vi "Header Footer Alignment.vi"(3 "H/F Alignment":T1) -> (0 "Vertical Alignement":T2, 1 "Horizontal Alignment":T3)   [LabVIEW 2012]
doc: "Version 1.0\nDeveloped by Jean-Marc Simard\nCopyright © 2010, Exaprom Inc.\nAll rights reserved.\nLicense: BSD\n\nWith iTextSharp 4.1.6 (http://itextsharp.sourceforge.net)\nunder Mozilla Public License Version 1.1\n(http://www.mozilla.org/MPL/MPL-1.1.html)"
uses:
  Controls/Header footer horiz alignment.ctl
  Controls/Cell Vertical alignment.ctl
  Controls/H F Alignment.ctl
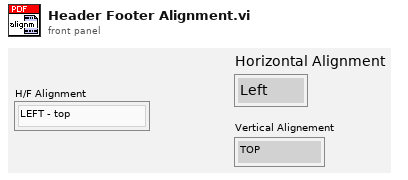
[diagram p1: front panel]
types:
  T1 = typedef "H F Alignment.ctl" = enum16{"LEFT - top", "LEFT - middle", "LEFT - bottom", "CENTER - top", "CENTER - middle", "CENTER - bottom", "RIGHT - top", "RIGHT - middle", "RIGHT - bottom", ""}
  T2 = typedef "Cell Vertical alignment.ctl" = enum16{"TOP", "MIDDLE", "BOTTOM"}
  T3 = typedef "Header footer horiz alignment.ctl" = enum16{"Left", "Center", "Right"}
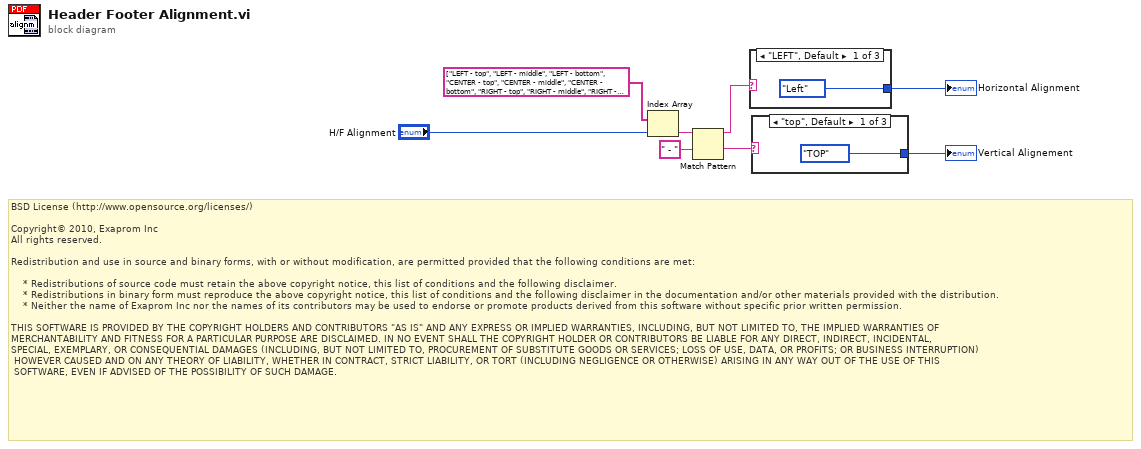
[diagram p0: block diagram]
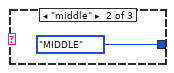
[diagram p2: hidden frame]
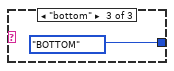
[diagram p3: hidden frame]
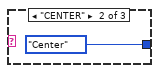
[diagram p4: hidden frame]
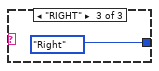
[diagram p5: hidden frame]
diagram:
  # "BSD License (http://www.opensource.org/licenses/)\n\nCopyright© 2010, Exaprom Inc\nAll rights reserved.\n\nRedistribution and use in source and binary forms, with or without modification, are permitted provided that the following conditions are met:\n\n    * Redistributions of source code must retain the above copyright notice, this list of conditions and the following disclaimer.\n    * Redistributions in binary form must reproduce the above copyright notice, this list of conditions and the following disclaimer in the documentation and/or other materials provided with the distribution.\n    * Neither the name of Exaprom Inc nor the names of its contributors may be used to endorse or promote products derived from this software without specific prior written permission.\n\nTHIS SOFTWARE IS PROVIDED BY THE COPYRIGHT HOLDERS AND CONTRIBUTORS \"AS IS\" AND ANY EXPRESS OR IMPLIED WARRANTIES, INCLUDING, BUT NOT LIMITED TO, THE IMPLIED WARRANTIES OF \nMERCHANTABILITY AND FITNESS FOR A PARTICULAR PURPOSE ARE DISCLAIMED. IN NO EVENT SHALL THE COPYRIGHT HOLDER OR CONTRIBUTORS BE LIABLE FOR ANY DIRECT, INDIRECT, INCIDENTAL,\nSPECIAL, EXEMPLARY, OR CONSEQUENTIAL DAMAGES (INCLUDING, BUT NOT LIMITED TO, PROCUREMENT OF SUBSTITUTE GOODS OR SERVICES; LOSS OF USE, DATA, OR PROFITS; OR BUSINESS INTERRUPTION)\n HOWEVER CAUSED AND ON ANY THEORY OF LIABILITY, WHETHER IN CONTRACT, STRICT LIABILITY, OR TORT (INCLUDING NEGLIGENCE OR OTHERWISE) ARISING IN ANY WAY OUT OF THE USE OF THIS\n SOFTWARE, EVEN IF ADVISED OF THE POSSIBILITY OF SUCH DAMAGE."
  n1 = Index Array(array=string[] ["LEFT - top", "LEFT - middle", "LEFT - bottom", "CENTER - top", "CENTER - middle", "CENTER - bottom", "RIGHT - top", "RIGHT - middle", "RIGHT - bottom", ""] ("Strings []"), index="H/F Alignment") -> (element=w8:string)
  n2 = Match Pattern(string=w8, regular expression=" - ") -> (before substring=w6:string, after substring=w5:string)  [unwired: 3 out]
  n3 = case shown="\"LEFT\", Default" w6 {
    tunnel: [Header_footer_horiz_alignment."Left" ("Alignment") Header_footer_horiz_alignment."Center" ("Alignment") Header_footer_horiz_alignment."Right" ("Alignment")] -> w3
    frame "LEFT", Default {
    }
    frame "CENTER" {
    }
    frame "RIGHT" {
    }
  }
  "Horizontal Alignment" <- w3
  n4 = case shown="\"top\", Default" w5 {
    tunnel: [Cell_Vertical_alignment."TOP" ("Vertical Alignement") Cell_Vertical_alignment."MIDDLE" ("Vertical Alignement") Cell_Vertical_alignment."BOTTOM" ("Vertical Alignement")] -> w2
    frame "top", Default {
    }
    frame "middle" {
    }
    frame "bottom" {
    }
  }
  "Vertical Alignement" <- w2
